vi "Power_Supply_GUI Server.vi"(8 "error in (no error)":errorcluster, 11 "Power_Supply Virtual in":refnum<class "Power_Supply Virtual.lvclass">) -> (0 "error out":errorcluster, 3 "Power_Supply Virtual out":refnum<class "Power_Supply Virtual.lvclass">)   [LabVIEW 2018, in "Power_Supply Virtual.lvclass"]
uses:
  Power_Supply Virtual.lvclass
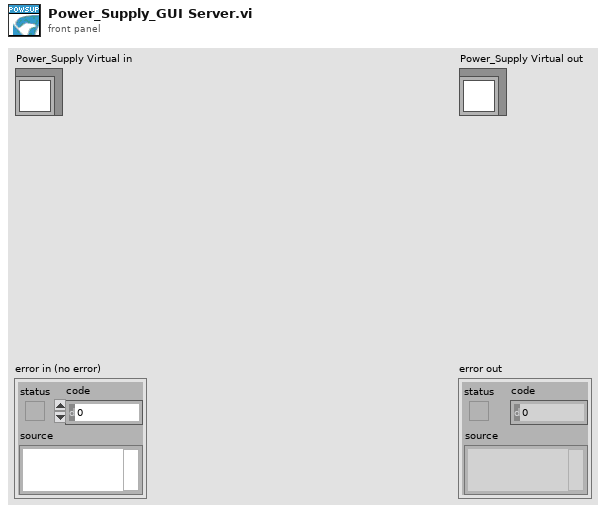
[diagram p1: front panel]
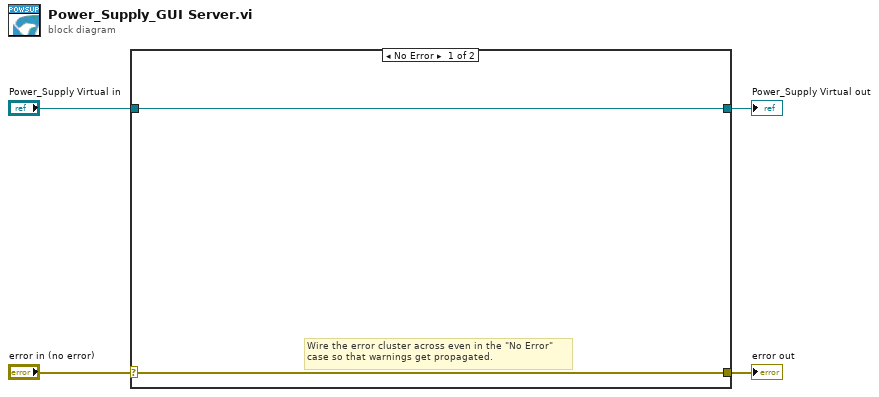
[diagram p0: block diagram]
diagram:
  n1 = case shown="No Error" "error in (no error)" {
    selector: "error in (no error)" -> [w5 w8]
    tunnel: [w5 w8] -> w3
    tunnel: [w6 w7] -> w1
    tunnel: "Power_Supply Virtual in" -> [w6 w7]
    frame No Error {
      # "Wire the error cluster across even in the \"No Error\"\ncase so that warnings get propagated."
    }
    frame Error {
    }
  }
  "error out" <- w3
  "Power_Supply Virtual out" <- w1
